vi "subsystem with sine wave.vi"(11 "frequency":dbl=0.5) -> (3 "Output":waveform(dbl)(graph)={"t0"=timestamp(9343.2 s since 1904-01-01), "dt"=1.0, "Y"=[0.2633720690985406]})   [LabVIEW 2011]
doc: "This subsystem produces a sine signal. When the VI on the local host runs, the Read/Write Model Parameters function in that VI sets the amplitude of the signal."
uses:
  <vilib>/Simulation/Implementation/Shared/SIMSCR Execution Mode.ctl
  <vilib>/Simulation/Scripting/Companion Diagram/SimConfigNode/SimParams.ctl
  <vilib>/Simulation/Scripting/Companion Diagram/SimConfigNode/_simSolvers.ctl
  <vilib>/Platform/TimedLoop/XDataNode/timing_clust.ctl
  <vilib>/Platform/TimedLoop/XDataNode/nitl_modes.ctl
  <vilib>/Platform/TimedLoop/XDataNode/wakeup.ctl
  <vilib>/Simulation/Param Hierarchy/Typedefs/SIMPH Param Control Actions.ctl
  <vilib>/Simulation/Implementation/Shared/NILVSim_FinishedLate.vi
  <vilib>/Simulation/DataSources/Implementation/NILVSim Sine Wave.llb/SIM Sine Wave (scalar).vi
  <vilib>/Simulation/SignalDisplay/Implementation/NILVSim Time Waveform.llb/SIM Time Waveform (scalar).vi
  <vilib>/Simulation/Implementation/Shared/NILVSim_Manager.vi
  <vilib>/Simulation/Implementation/Shared/NILVSim_ParamChanged.vi
  <vilib>/Simulation/Implementation/Shared/NILVSim_FinalizeModel.vi
  <vilib>/Simulation/Utility/Implementation/NILVSim Get Time and IsAcceptedStep.vi
  <vilib>/Simulation/Implementation/Shared/SIM Unbundle Sim Info.vi
  <vilib>/Simulation/Implementation/Shared/NILVSim_GetModelError.vi
  <vilib>/Simulation/Implementation/Shared/SIM SimErrorHandler.vi
  <vilib>/Simulation/Implementation/Shared/SIM Bundle Sim Info.vi
  <vilib>/Simulation/Implementation/Shared/NILVSim_Initialize.vi
  <vilib>/Simulation/Scripting/Companion Diagram/SimConfigNode/SimDog.xnode
  <vilib>/Platform/TimedLoop/XDataNode/XDataNode.xnode
  <vilib>/Simulation/Implementation/XNodeFramework/SimXNode/SimX.xnode
  <vilib>/Platform/TimedLoop/XDataNode/XDNodeRunTimeDep.lvlib
  <vilib>/Simulation/Implementation/Shared/NI_SIM_Implementation.lvlib
panel:
  # "This subsystem produces a sine signal. When the VI on the local host runs, the \nRead/Write Model Parameters function sets the amplitude of the signal."
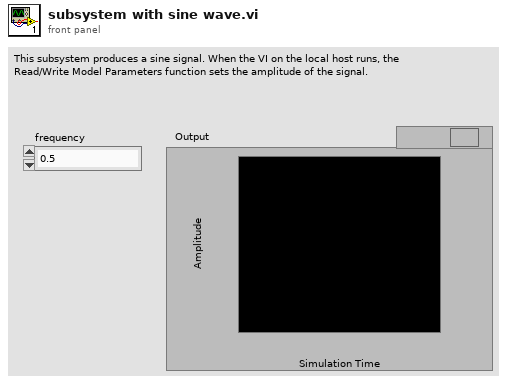
[diagram p1: front panel]
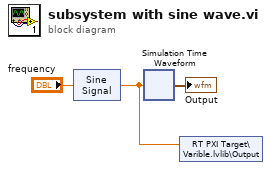
[diagram p0: block diagram]
diagram:
  n1 = xnode "Sine Signal"("frequency"="frequency") -> ("output"=w1:dbl)  [unwired: 5 in]
  n2 = xnode ("Simulation Time Waveform")("Value"=w1) -> ("Waveform Chart"=→"Output":waveform(dbl))  [unwired: 1 in]
  n3 = shared-variable "RT PXI Target\\Varible.lvlib\\Output"(w1) -> ()  [unwired: 1 in, 1 out]
